vi "DetectNewKbHit.vi"(7 "SelectKb":T2, 8 "error in":errorcluster) -> (0 "error out":errorcluster, 2 "NewKey":bool[](array[boolean]), 3 "keys pressed":T1(array[ring]))   [LabVIEW 2022 SP3]
uses:
  SelectKb.ctl
  <vilib>/Utility/inputDevices.llb/keyboardAcquire.vi
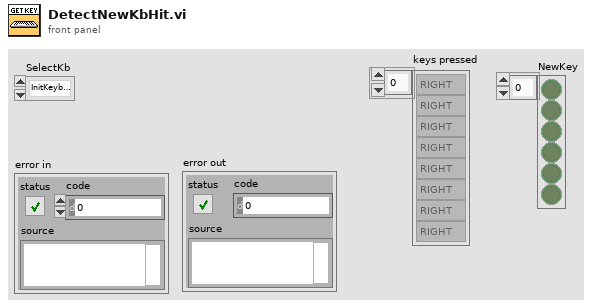
[diagram p1: front panel]
types:
  T1 = enum16{"0", "1", "2", "3", "4", "5", "6", "7", "8", "9", "A", "B", "C", "D", "E", "F", "G", "H", "I", "J", "K", "L", "M", "N", "O", "P", "Q", "R", "S", "T", "U", "V", "W", "X", "Y", "Z", "F1", "F2", "F3", "F4", "F5", "F6", "F7", "F8", "F9", "F10", "F11", "F12", "F13", "F14", "F15", "ADD", "BACK", "BACKSLASH", "CAPITAL", "COMMA", "DECIMAL", "DELETE", "DIVIDE", "DOWN", "END", "EQUALS", "ESCAPE", "GRAVE (`)", "HOME", "INSERT", "LBRACKET", "LCONTROL", "LEFT", "L ALT", "LSHIFT", "LWIN", "MINUS", "MULTIPLY", "NEXT", "NUMLOCK", "NUMPAD_0", "NUMPAD_1", "NUMPAD_2", "NUMPAD_3", "NUMPAD_4", "NUMPAD_5", "NUMPAD_6", "NUMPAD_7", "NUMPAD_8", "NUMPAD_9", "PAUSE", "PERIOD", "PRIOR (PG UP)", "RBRACKET", "RCONTROL", "RETURN", "RIGHT", "R ALT", "RSHIFT", "RWIN", "SCROLL", "SEMICOLON", "SLASH", "SPACE", "SUBTRACT", "TAB", "UP", "ENTER (num pad)", "' (quote)"}[]
  T2 = typedef "SelectKb.ctl" = enum16{"InitKeyboard", "GetPressedKeys"}
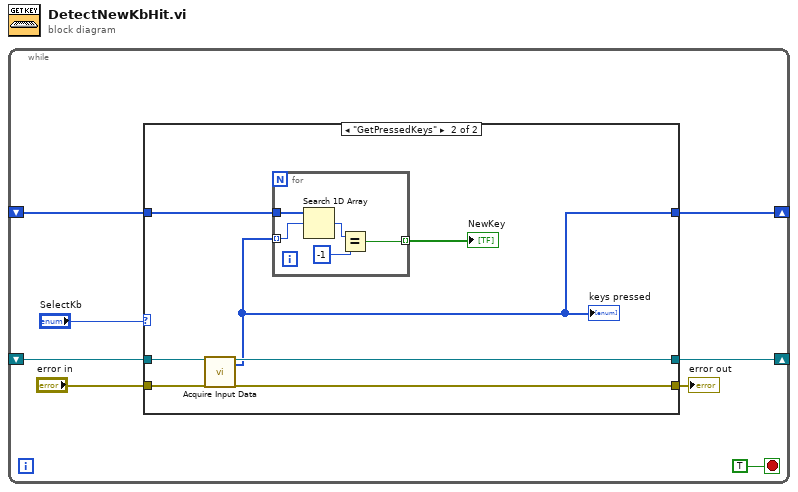
[diagram p0: block diagram]
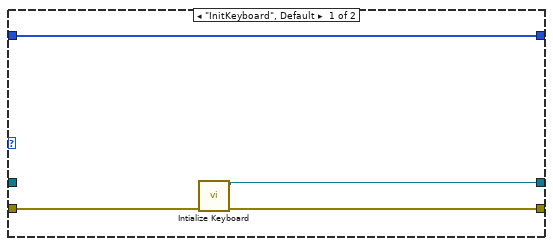
[diagram p2: hidden frame]
diagram:
  n1 = while {
    shift-right: [w5] -> _
    shift-left: _ -> [w3]
    shift-right: [w2] -> _
    shift-left: _ -> [w1]
    stop <- TRUE stop-if-true
    n2 = case shown="\"GetPressedKeys\"" "SelectKb" {
      tunnel: "error in" -> [w11 w19]
      tunnel: [w12 w18] -> w4
      tunnel: [w10 w16] -> w5
      tunnel: w3 -> [_ w17]
      tunnel: [w9 w14] -> w2
      tunnel: w1 -> [w9 w15]
      frame "InitKeyboard", Default {
        n3 = call <vilib>:"Intialize Keyboard.vi"("error in (no error)"=w11) -> ("error out"=w12:errorcluster, "device ID"=w10:refnum<k1>)  [unwired: 9 in]
      }
      frame "GetPressedKeys" {
        n4 = call-poly <vilib>:"Acquire Input Data.vi"("device ID"=w17, "error in (no error)"=w19) -> ("device ID"=w16:refnum<k1>, "keys pressed"=w14:T1, "error out"=w18:errorcluster)  [unwired: 15 in]
        "keys pressed" <- w14
        n5 = for {
          tunnel: w14 -> [w23] mode=indexing
          tunnel: w15 -> [w24]
          tunnel: [w20] -> w13 mode=indexing
          n6 = Search 1D Array(1D array=w24, element=w23) -> (index of element=w22:i32)  [unwired: 1 in]
          n7 = Equal?(x=w22, y=-1) -> (x = y?=w20:bool)
        }
        "NewKey" <- w13
      }
    }
    "error out" <- w4
  }
